vi "Scan last shot data.vi"(8 "error in (no error)":errorcluster) -> (0 "error out":errorcluster)   [LabVIEW 2015]
uses:
  Shot data.ctl
  <vilib>/Utility/config.llb/NI_LVConfig.lvlib
  <vilib>/Utility/config.llb/Write Key (Boolean).vi
panel:
  out "resulting string":string="Shot number = 33\nTime = 12:20:00.259 PM 1/26/2012\nMagnet ID = \"sdqwde\"\nUser = \"sAXWCD\"\nCell number = 1\nRequested field = 65.000000\nField direction = \"UP\"\nNumber of bank frames = 8\nCrowbar resistance, mOhm = 25.000000\nMagnet resistance, mOhm = 35.000000\nCharger voltage, kV = 9.000000\nFrame voltage, kV = 10.000000"
  out "output 1":timestamp
  out "date/time string":string
  out "time string":string
  out "date string":string
  out "Array":u32[](array[numeric])
  out "Shot data elements":string[](array[string])=["Shot number", "Time", "Magnet ID", "User", "Cell number", "Requested field", "Field direction", "Number of bank frames", "Crowbar resistance, mOhm", "Magnet resistance, mOhm", "Charger voltage, kV", "Frame voltage, kV"]
  in  "Shot data":T1={"Shot number"=33, "Time"=timestamp(3410450400.259543 s since 1904-01-01), "Magnet ID"="sdqwde", "User"="sAXWCD", "Cell number"=1, "Requested field"=65.0, "Field direction"="UP", "Number of bank frames"=8, "Crowbar resistance, mOhm"=25.0, "Magnet resistance, mOhm"=35.0, "Charger voltage, kV"=9.0, "Frame voltage, kV"=10.0}
  in  "File path":path=path "C:/data/LastShot.txt"
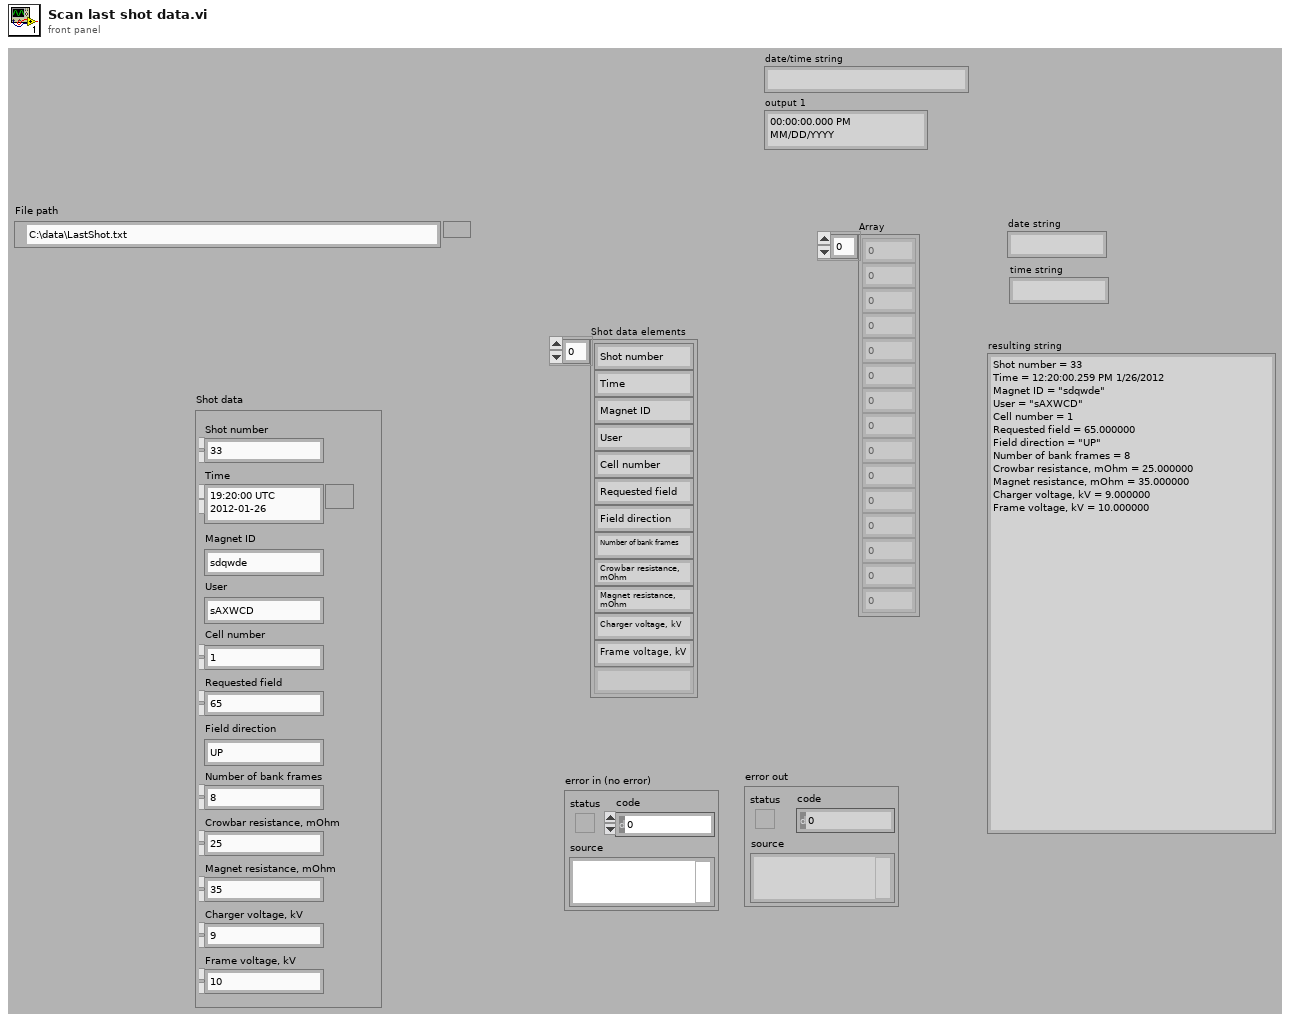
[diagram p1: front panel]
types:
  T1 = typedef "Shot data.ctl" = cluster{"Shot number":i32, "Time":timestamp, "Magnet ID":string, "User":string, "Cell number":i32, "Requested field":dbl, "Field direction":string, "Number of bank frames":i32, "Crowbar resistance, mOhm":dbl, "Magnet resistance, mOhm":dbl, "Charger voltage, kV":dbl, "Frame voltage, kV":dbl}
  T2 = cluster{"Shot data elements[0]":string, "Shot data elements[1]":string, "Shot data elements[2]":string, "Shot data elements[3]":string, "Shot data elements[4]":string, "Shot data elements[5]":string, "Shot data elements[6]":string, "Shot data elements[7]":string, "Shot data elements[8]":string, "Shot data elements[9]":string, "Shot data elements[10]":string, "Shot data elements[11]":string}
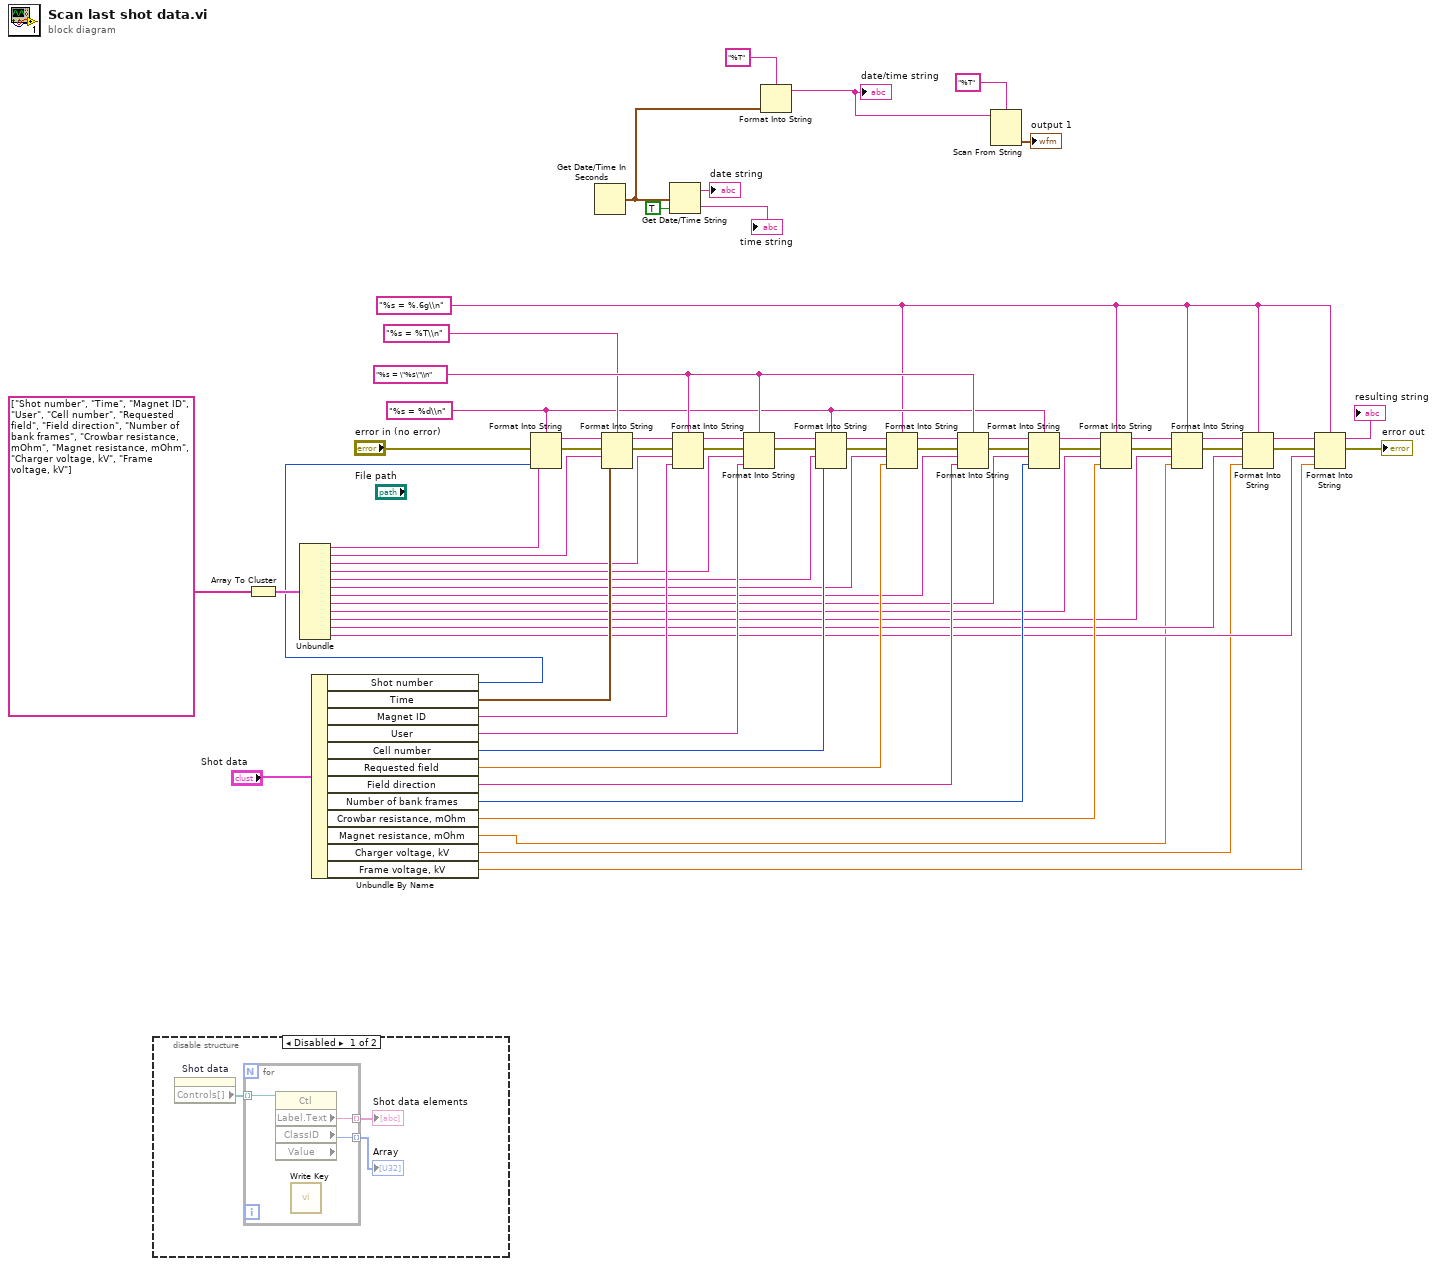
[diagram p0: block diagram]
diagram:
  w4 = "%s = %.6g\\n" ("format string")
  w31 = "%s = \"%s\"\\n" ("format string")
  w23 = "%s = %d\\n" ("format string")
  n1 = disable-structure shown="Disabled" {
    frame Disabled {
      n2 = property on="Shot data" class="Clust (strict)"() -> ("Controls[]"=w67:refnum<vi>[])  [unwired: 2 in, 2 out]
      n3 = for {
        tunnel: w67 -> [w70] mode=indexing
        tunnel: [w69] -> w66 mode=indexing
        tunnel: [w68] -> w65 mode=indexing
        n4 = property class="Ctl" props=["Label", "Text", "ClassID", "Value"](reference=w70) -> ("Label.Text"=w69:string, "ClassID"=w68:u32)  [unwired: 1 in, 3 out]
        n5 = call-poly <vilib>:"Write Key.vi"() -> ()  [unwired: 9 in, 3 out]
      }
      "Shot data elements" <- w66
      "Array" <- w65
    }
    frame Enabled {
    }
  }
  n6 = Array To Cluster(array=string[] ["Shot number", "Time", "Magnet ID", "User", "Cell number", "Requested field", "Field direction", "Number of bank frames", "Crowbar resistance, mOhm", "Magnet resistance, mOhm", "Charger voltage, kV", "Frame voltage, kV"] ("Shot data elements")) -> (cluster=w63:T2)
  n7 = Unbundle(w63) -> ("Shot data elements[0]"=w53:string, "Shot data elements[1]"=w51:string, "Shot data elements[2]"=w46:string, "Shot data elements[3]"=w44:string, "Shot data elements[4]"=w37:string, "Shot data elements[5]"=w33:string, "Shot data elements[6]"=w29:string, "Shot data elements[7]"=w25:string, "Shot data elements[8]"=w20:string, "Shot data elements[9]"=w10:string, "Shot data elements[10]"=w9:string, "Shot data elements[11]"=w8:string)
  n8 = Unbundle By Name("Shot data") -> ("Shot number"=w52:i32, "Time"=w49:timestamp, "Magnet ID"=w45:string, "User"=w43:string, "Cell number"=w36:i32, "Requested field"=w32:dbl, "Field direction"=w26:string, "Number of bank frames"=w24:i32, "Crowbar resistance, mOhm"=w19:dbl, "Magnet resistance, mOhm"=w5:dbl, "Charger voltage, kV"=w6:dbl, "Frame voltage, kV"=w7:dbl)
  n9 = Format Into String(format string=w23, error in="error in (no error)", w53, w52) -> (resulting string=w50:string, error out=w48:errorcluster)  [unwired: 1 in]
  n10 = Get Date/Time In Seconds() -> (seconds since 1Jan1904=w55:timestamp)
  n11 = Format Into String(format string="%s = %T\\n", initial string=w50, error in=w48, w51, w49) -> (resulting string=w41:string, error out=w47:errorcluster)
  n12 = Get Date/Time String(seconds (now)=w55, want seconds? (F)=TRUE) -> (date string=→"date string":string, time string=→"time string":string)  [unwired: 1 in]
  n13 = Format Into String(format string=w31, initial string=w41, error in=w47, w46, w45) -> (resulting string=w40:string, error out=w42:errorcluster)
  n14 = Format Into String(format string=w31, initial string=w40, error in=w42, w44, w43) -> (resulting string=w38:string, error out=w39:errorcluster)
  n15 = Format Into String(format string="%T", w55) -> (resulting string=w54:string)  [unwired: 2 in, 1 out]
  "date/time string" <- w54
  n16 = Format Into String(format string=w23, initial string=w38, error in=w39, w37, w36) -> (resulting string=w35:string, error out=w34:errorcluster)
  n17 = Format Into String(format string=w4, initial string=w35, error in=w34, w33, w32) -> (resulting string=w30:string, error out=w28:errorcluster)
  n18 = Format Into String(format string=w31, initial string=w30, error in=w28, w29, w26) -> (resulting string=w21:string, error out=w22:errorcluster)
  n19 = Scan From String(format string="%T", input string=w54) -> (output 1=→"output 1":timestamp)  [unwired: 3 in, 3 out]
  n20 = Format Into String(format string=w23, initial string=w21, error in=w22, w25, w24) -> (resulting string=w18:string, error out=w17:errorcluster)
  n21 = Format Into String(format string=w4, initial string=w18, error in=w17, w20, w19) -> (resulting string=w16:string, error out=w13:errorcluster)
  n22 = Format Into String(format string=w4, initial string=w16, error in=w13, w10, w5) -> (resulting string=w15:string, error out=w14:errorcluster)
  n23 = Format Into String(format string=w4, initial string=w15, error in=w14, w9, w6) -> (resulting string=w11:string, error out=w12:errorcluster)
  n24 = Format Into String(format string=w4, initial string=w11, error in=w12, w8, w7) -> (resulting string=→"resulting string":string, error out=→"error out":errorcluster)
